vi "Get Selected Project Path.vi"(8 "error in":errorcluster, 11 "Project Name":string) -> (0 "error out":errorcluster, 3 "Project Path":path)   [LabVIEW 2019, in "Panther Dashboard.lvlib"]
uses:
  Panther Dashboard.lvlib
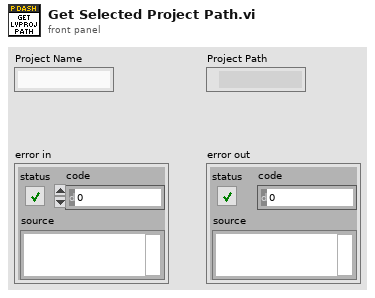
[diagram p1: front panel]
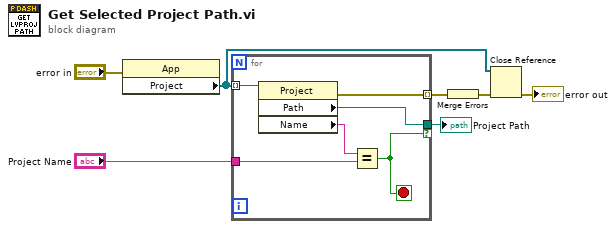
[diagram p0: block diagram]
diagram:
  n1 = property class="App"(error in="error in") -> ("Project"=w4:refnum<vi>[])  [unwired: 1 in, 2 out]
  n2 = for {
    tunnel: w4 -> [w12] mode=indexing
    tunnel: [w8] -> w1 if=w11
    tunnel: [w13] -> w3 mode=indexing
    tunnel: "Project Name" -> [w10]
    stop <- w11 stop-if-true
    n3 = property class="Project"(reference=w12) -> (error out=w13:errorcluster, "Path"=w8:path, "Name"=w9:string)  [unwired: 1 in, 1 out]
    n4 = Equal?(x=w9, y=w10) -> (x = y?=w11:bool)
  }
  "Project Path" <- w1
  n5 = Merge Errors(w3) -> (w5:errorcluster)
  n6 = Close Reference(reference=w4, error in (no error)=w5) -> (error out=→"error out":errorcluster)
